vi "append_return_data.vi"(11 "Return Data":string) -> ()   [LabVIEW 2013, in "Experiment.lvclass"]
uses:
  Experiment.lvclass
  Globals.vi
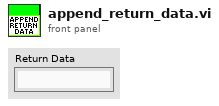
[diagram p1: front panel]
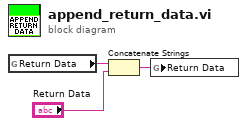
[diagram p0: block diagram]
diagram:
  n1 = global read "Globals.vi" "Return Data"() -> (w3:string)
  n2 = Concatenate Strings(w3, "Return Data") -> (w1:string)
  n3 = global write "Globals.vi" "Return Data"(w1) -> ()
